vi "Parse Arguments.vi"(7 "Label Marker (-)":string="-", 8 "error in (no error)":errorcluster, 10 "Arguments":string[](array[string]), 11 "Option Set in":refnum<class "Option Set.lvclass">) -> (0 "error out":errorcluster, 1 "Missing Options":bool, 3 "Option Set out":refnum<class "Option Set.lvclass">, 4 "Missing Option Keys":string[](array[string]))   [LabVIEW 2011, in "Option Parser.lvlib" / "Option Set.lvclass"]
doc: "Parses the incoming arguments. After this VI you can get values for options and trailing arguments (arguments not attached to an option).\n\n<b>Label Marker</b> defines the string that comes in front of an option label. e.g. if the Label Marker is - and the label is option we will look for -option as an argument."
uses:
  Option Set.lvclass
  Option Set.lvclass/Option Set.ctl
  Option Class/Option.lvclass/Option.ctl
  <vilib>/regexp/Match Regular Expression.xnode
  Option Class/Option.lvclass
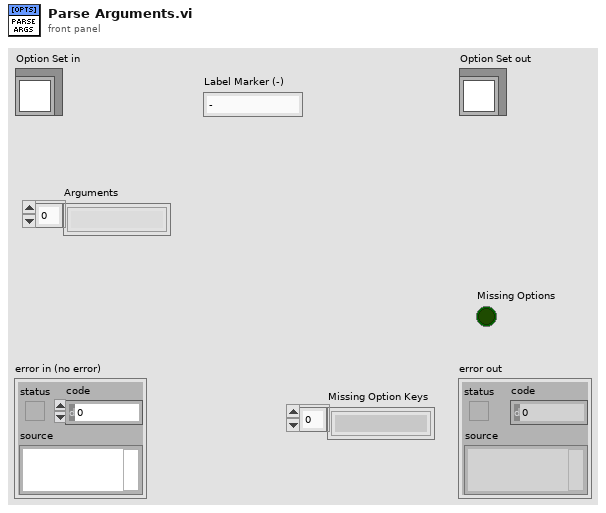
[diagram p1: front panel]
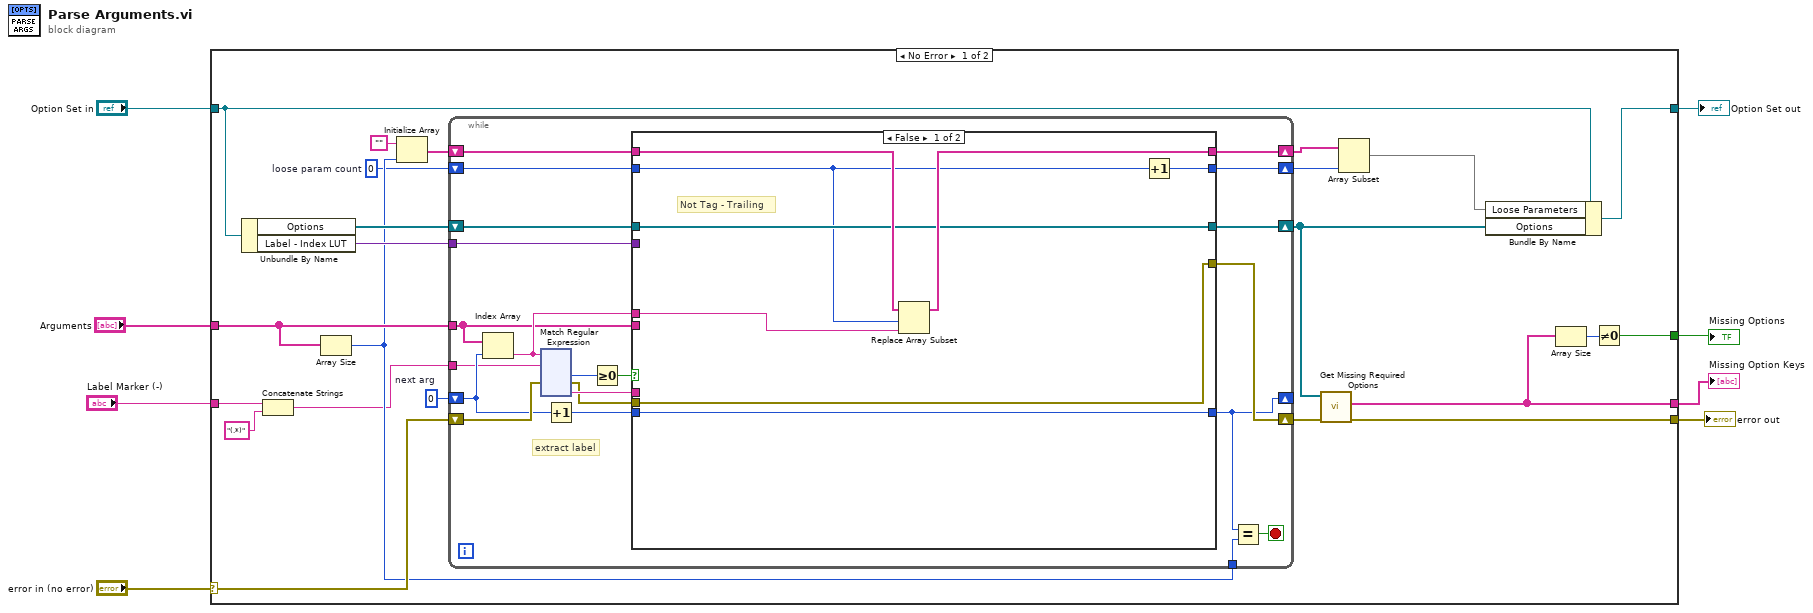
[diagram p0: block diagram]
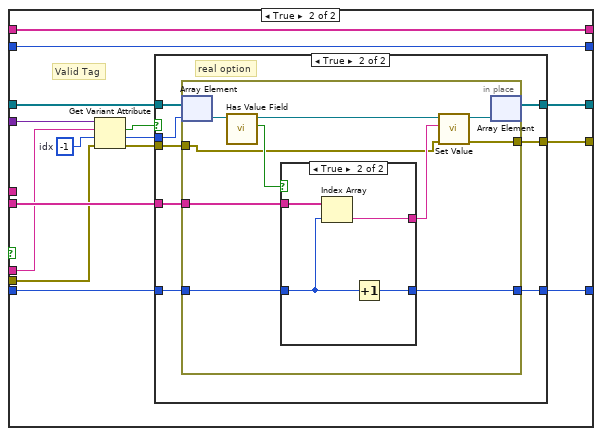
[diagram p2: hidden frame]
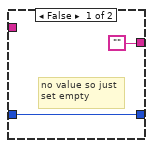
[diagram p4: hidden frame]
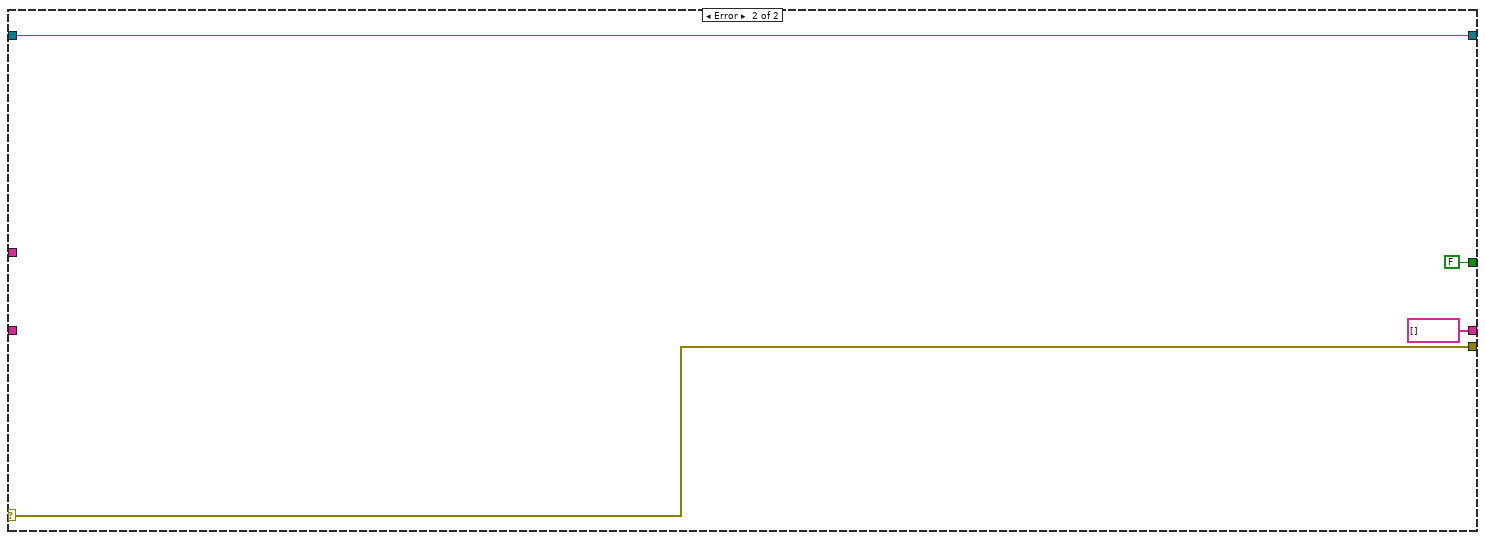
[diagram p5: hidden frame]
diagram:
  n1 = case shown="No Error" "error in (no error)" {
    selector: "error in (no error)" -> [w30 w219]
    tunnel: [w13 w219] -> w7
    tunnel: [w27 w218] -> w5
    tunnel: "Option Set in" -> [w26 w218]
    tunnel: "Arguments" -> [w25 _]
    tunnel: "Label Marker (-)" -> [w16 _]
    tunnel: [w11 string[] [] ("Missing Keys")] -> w2
    tunnel: [w9 FALSE] -> w1
    frame No Error {
      w20 = 0  # loose param count
      w31 = 0  # next arg
      n2 = Unbundle By Name(w26) -> ("Options"=w29:refnum<class "Option.lvclass">[], "Label - Index LUT"=w28:variant)
      n3 = Concatenate Strings(w16, "(.*)" ("string")) -> (w14:string)
      n4 = Array Size(array=w25) -> (size(s)=w22:i32)
      n5 = Initialize Array("", w22) -> (w24:string[])
      n6 = while {
        tunnel: w25 -> [w46]
        shift-right: [w36] -> _
        shift-left: w31 -> [w49]
        shift-right: [w45] -> w21
        shift-left: w24 -> [w44]
        shift-right: [w39] -> w12
        shift-left: w29 -> [w40]
        tunnel: w28 -> [w43]
        shift-right: [w38] -> w17
        shift-left: w30 -> [w52]
        tunnel: w22 -> [w35]
        shift-right: [w34] -> w18
        shift-left: w20 -> [w33]
        tunnel: w14 -> [w32]
        stop <- w37 stop-if-true
        # "extract label"
        n7 = Index Array(array=w46, index=w49) -> (element=w47:string)
        n8 = xnode "Match Regular Expression"("input string"=w47, "regular expression"=w32, "error in"=w52) -> ("offset past match"=w51:i32, "error out"=w41:errorcluster, "submatch 1"=w42:string)  [unwired: 3 in, 3 out]
        n9 = Increment(x=w49) -> (x+1=w48:i32)
        n10 = Greater Or Equal To 0?(x=w51) -> (x >= 0?=w50:bool)
        n11 = case shown="False" w50 {
          tunnel: w48 -> [w60 w73]
          tunnel: [w60 w72] -> w36
          tunnel: w47 -> [w55 _]
          tunnel: w46 -> [_ w74]
          tunnel: [w59 w75] -> w45
          tunnel: w44 -> [w58 w75]
          tunnel: w43 -> [_ w71]
          tunnel: w42 -> [_ w70]
          tunnel: w41 -> [w56 w68]
          tunnel: w40 -> [w57 w67]
          tunnel: [w57 w66] -> w39
          tunnel: [w56 w63] -> w38
          tunnel: [w53 w61] -> w34
          tunnel: w33 -> [w54 w61]
          frame False {
            # "Not Tag - Trailing"
            n12 = Replace Array Subset(array=w58, new element=w55, index=w54) -> (w59:string[])
            n13 = Increment(x=w54) -> (x+1=w53:i32)
          }
          frame True {
            w69 = -1  # idx
            # "Valid Tag"
            n14 = Get Variant Attribute(Variant=w71, name=w70, default value (empty Variant)=w69, error in=w68) -> (found=w62:bool, value=w65:i32, error out=w64:errorcluster)  [unwired: 1 out]
            n15 = case shown="True" w62 {
              tunnel: w74 -> [_ w86]
              tunnel: w73 -> [w78 w85]
              tunnel: [w78 w84] -> w72
              tunnel: w67 -> [w76 w83]
              tunnel: [w76 w82] -> w66
              tunnel: w65 -> [_ w81]
              tunnel: w64 -> [w77 w80]
              tunnel: [w77 w79] -> w63
              frame False {
              }
              frame True {
                # "real option"
                n16 = in-place {
                  in-place-border: w86 -> [w96]
                  in-place-border: w85 -> [w95]
                  in-place-border: [w94] -> w84
                  in-place-border: w80 -> [w87]
                  in-place-border: [w90] -> w79
                  n17 = in-place-array #1(w83, w81) -> (w93:refnum<class "Option.lvclass">)
                  n18 = call "Has Value Field.vi"("Option in"=w93) -> ("Has Value Field"=w89:bool, "Option out"=w91:refnum<class "Option.lvclass">)  [unwired: 9 in]
                  n19 = case shown="True" w89 {
                    tunnel: w96 -> [_ w102]
                    tunnel: w95 -> [w98 w101]
                    tunnel: [w98 w100] -> w94
                    tunnel: ["" w99] -> w88
                    frame False {
                      # "no value so just\nset empty"
                    }
                    frame True {
                      n20 = Index Array(array=w102, index=w101) -> (element=w99:string)
                      n21 = Increment(x=w101) -> (x+1=w100:i32)
                    }
                  }
                  n22 = call "Set Value.vi"("error in (no error)"=w87, "Value"=w88, "Option in"=w91) -> ("error out"=w90:errorcluster, "Option out"=w92:refnum<class "Option.lvclass">)  [unwired: 7 in]
                  n23 = in-place-array #1(w92) -> (w82:refnum<class "Option.lvclass">[])  [unwired: 1 out]
                }
              }
            }
          }
        }
        n24 = Equal?(x=w36, y=w35) -> (x = y?=w37:bool)
      }
      n25 = call "Get Missing Required Options.vi"("error in (no error)"=w17, "Options"=w12) -> ("error out"=w13:errorcluster, "Missing Keys"=w11:string[])  [unwired: 8 in]
      n26 = Array Subset(array=w21, length=w18) -> (w19:string[])  [unwired: 1 in]
      n27 = Bundle By Name(cluster=w26, "Loose Parameters"=w19, "Options"=w12) -> (w27:refnum<class "Option Set.lvclass">)
      n28 = Array Size(array=w11) -> (size(s)=w10:i32)
      n29 = Not Equal To 0?(x=w10) -> (x != 0?=w9:bool)
    }
    frame Error {
    }
  }
  "error out" <- w7
  "Option Set out" <- w5
  "Missing Option Keys" <- w2
  "Missing Options" <- w1
